vi "VI Operation.vi"(8 "error in (no error)":errorcluster, 9 "VI Name":string, 10 "Operation":string, 11 "Model in":refnum<class "Model.lvclass">) -> (0 "error out":errorcluster, 3 "Model out":refnum<class "Model.lvclass">)   [LabVIEW 2015, in "Model.lvlib" / "Model.lvclass"]
uses:
  Model.lvclass
  Model Messages/Edit Icon Msg/Edit Icon Msg.lvclass
  <vilib>/ActorFramework/Actor/Actor.lvclass
  Model Messages/Save All VIs Msg/Save All VIs Msg.lvclass
  Model Messages/Remove VI Msg/Remove VI Msg.lvclass
  Model Messages/Configure VI Analyzer Msg/Configure VI Analyzer Msg.lvclass
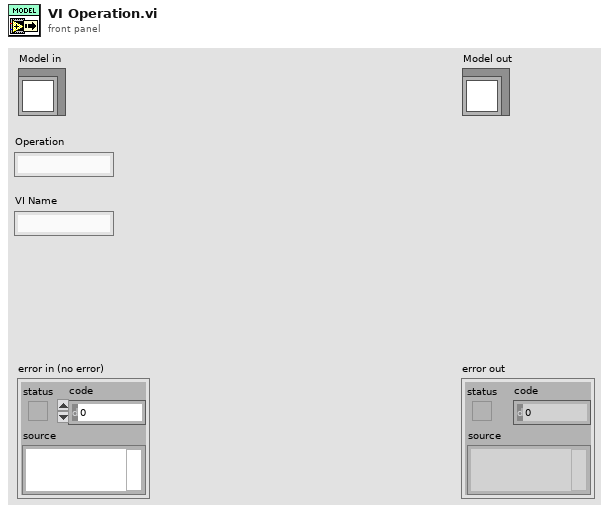
[diagram p1: front panel]
types:
  T1 = enum32{"Invalid", "Standard", "Closed", "Hidden", "Minimized", "Maximized"}
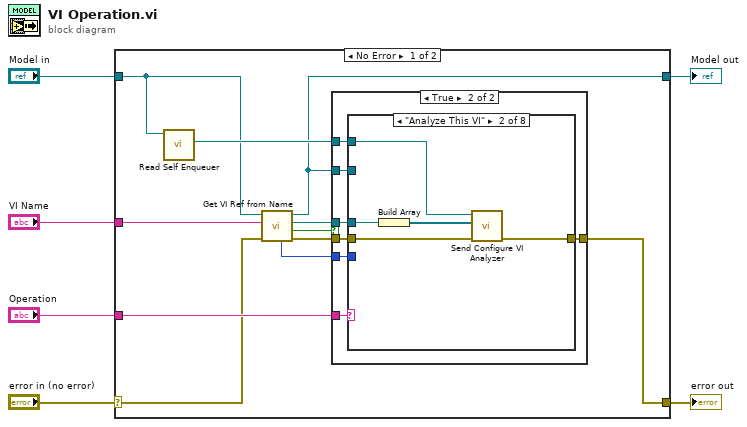
[diagram p0: block diagram]
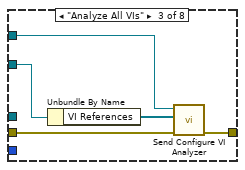
[diagram p4: hidden frame]
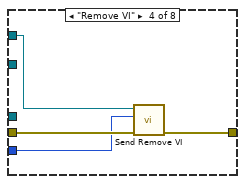
[diagram p5: hidden frame]
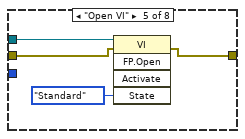
[diagram p6: hidden frame]
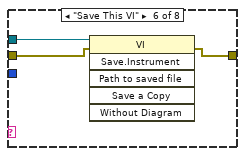
[diagram p7: hidden frame]
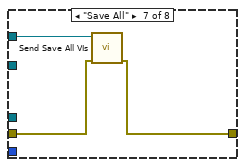
[diagram p8: hidden frame]
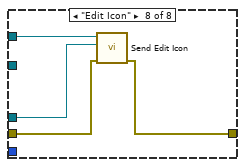
[diagram p9: hidden frame]
diagram:
  n1 = case shown="No Error" "error in (no error)" {
    selector: "error in (no error)" -> [w11 w56]
    tunnel: [w9 w56] -> w5
    tunnel: [w7 w55] -> w3
    tunnel: "Model in" -> [w15 w55]
    tunnel: "VI Name" -> [w14 _]
    tunnel: "Operation" -> [w17 _]
    frame No Error {
      n2 = call <vilib>:"Read Self Enqueuer.vi"("Actor"=w15) -> ("Self Enqueuer"=w16:refnum<class "Message Enqueuer.lvclass">)  [unwired: 10 in]
      n3 = call "Get VI Ref from Name.vi"("error in (no error)"=w11, "VI Name"=w14, "Model in"=w15) -> ("error out"=w10:errorcluster, "Found?"=w12:bool, "VI Refnum"=w13:refnum<vi>, "Model out"=w7:refnum<class "Model.lvclass">, "Index"=w8:i32)  [unwired: 4 in]
      n4 = case shown="True" w12 {
        tunnel: w17 -> [_ w25]
        tunnel: w16 -> [_ w24]
        tunnel: w13 -> [_ w23]
        tunnel: w10 -> [w18 w22]
        tunnel: [w18 w21] -> w9
        tunnel: w8 -> [_ w20]
        tunnel: w7 -> [_ w19]
        frame False {
        }
        frame True {
          n5 = case shown="\"Analyze This VI\"" w25 {
            tunnel: w24 -> [_ w31 w34 w40 _ _ w50 w54]
            tunnel: w23 -> [_ w28 _ _ w43 w47 _ w53]
            tunnel: w22 -> [w26 w30 w35 w39 w42 w46 w49 w52]
            tunnel: [w26 w29 w36 w38 w41 w45 w48 w51] -> w21
            tunnel: w20 -> [_ _ _ w37 _ _ _ _]
            tunnel: w19 -> [_ _ w33 _ _ _ _ _]
            frame "False", Default {
            }
            frame "Analyze This VI" {
              n6 = Build Array(w28) -> (w27:refnum<vi>[])
              n7 = call "Send Configure VI Analyzer.vi"("error in (no error)"=w30, "VI References"=w27, "Message Enqueuer"=w31) -> ("error out"=w29:errorcluster)  [unwired: 7 in, 1 out]
            }
            frame "Analyze All VIs" {
              n8 = Unbundle By Name(w33) -> ("VI References"=w32:refnum<vi>[])
              n9 = call "Send Configure VI Analyzer.vi"("error in (no error)"=w35, "VI References"=w32, "Message Enqueuer"=w34) -> ("error out"=w36:errorcluster)  [unwired: 7 in, 1 out]
            }
            frame "Remove VI" {
              n10 = call "Send Remove VI.vi"("error in (no error)"=w39, "Index to remove"=w37, "Message Enqueuer"=w40) -> ("error out"=w38:errorcluster)  [unwired: 7 in, 1 out]
            }
            frame "Open VI" {
              n11 = invoke class="VI" method="FP.Open"(reference=w43, error in=w42, "State"=T1."Standard") -> (error out=w41:errorcluster)  [unwired: 2 in, 4 out]
            }
            frame "Save This VI" {
              n12 = invoke class="VI" method="Save.Instrument"(reference=w47, error in=w46) -> (error out=w45:errorcluster)  [unwired: 4 in, 5 out]
            }
            frame "Save All" {
              n13 = call "Send Save All VIs.vi"("error in (no error)"=w49, "Message Enqueuer"=w50) -> ("error out"=w48:errorcluster)  [unwired: 8 in, 1 out]
            }
            frame "Edit Icon" {
              n14 = call "Send Edit Icon.vi"("error in (no error)"=w52, "VI Refnum in"=w53, "Message Enqueuer"=w54) -> ("error out"=w51:errorcluster)  [unwired: 7 in, 1 out]
            }
          }
        }
      }
    }
    frame Error {
    }
  }
  "error out" <- w5
  "Model out" <- w3
